vi "LV SciSDK SPECTRUM.vi"(9 "Spectrum Handle In":T2) -> (1 "Spectrum Handle Out":T2, 2 "Spectrum Data Buffer Out":T1)   [LabVIEW 2021]
uses:
  SciSDK_Labview.lvlib
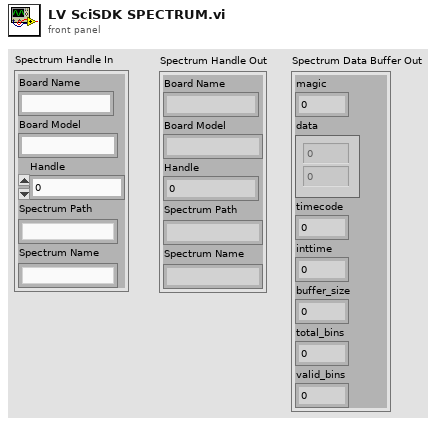
[diagram p1: front panel]
types:
  T1 = cluster{"magic":u32, "data":i32[], "timecode":u32, "inttime":u32, "buffer_size":u32, "total_bins":u32, "valid_bins":u32}
  T2 = cluster{"Board Name":string, "Board Model":string, "Handle":u64, "Spectrum Path":string, "Spectrum Name":string}
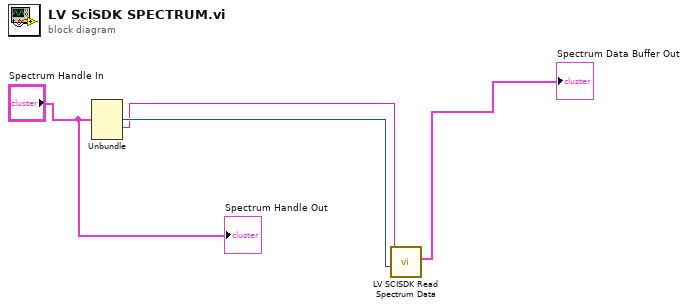
[diagram p0: block diagram]
diagram:
  n1 = Unbundle("Spectrum Handle In") -> ("Handle"=w3:u64, "Spectrum Path"=w2:string)  [unwired: 3 out]
  n2 = call "LV SCISDK Read Spectrum Data.vi"("Path"=w2, "handle"=w3) -> ("buffer out"=→"Spectrum Data Buffer Out":T1)  [unwired: 5 in, 3 out]
  "Spectrum Handle Out" <- "Spectrum Handle In"
